vi "Parse and Replace Strings for Downlink.vi"(9 "Input String":string) -> (2 "Output String":string)   [LabVIEW 2010]
doc: "This VI Replaces the string \"ProgramDisabled=YES\" with \"ProgramDisabled=0\" and replaces all instances of \"YES\" with \"1\", all instances of \"NO\" with \"0\". The resulting string is output to the Output String indicator."
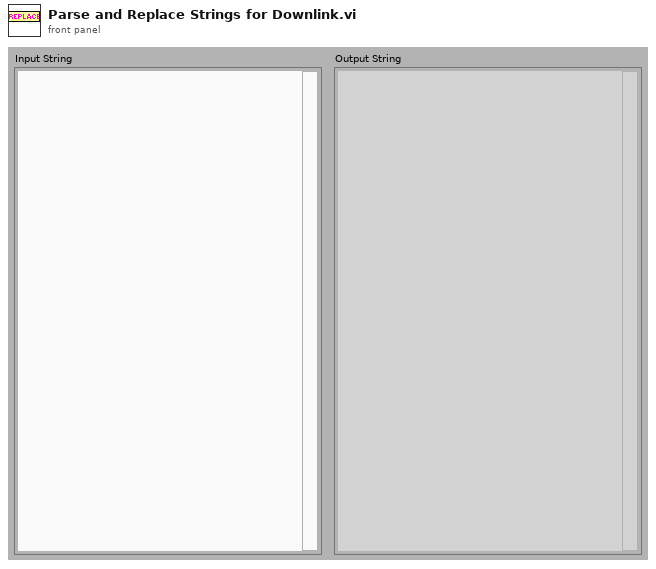
[diagram p1: front panel]
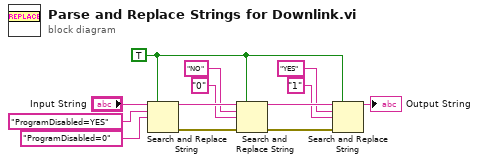
[diagram p0: block diagram]
diagram:
  w7 = TRUE ("replace all? (F)")
  n1 = Search and Replace String(replace all?=w7, input string="Input String", search string="ProgramDisabled=YES" ("regular expression"), replace string="ProgramDisabled=0" ("regular expression")) -> (result string=w13:string, error out=w6:errorcluster)  [unwired: 4 in, 2 out]
  n2 = Search and Replace String(replace all?=w7, input string=w13, search string="NO" ("regular expression"), replace string="0" ("regular expression"), error in=w6) -> (result string=w12:string, error out=w5:errorcluster)  [unwired: 3 in, 2 out]
  n3 = Search and Replace String(replace all?=w7, input string=w12, search string="YES" ("regular expression"), replace string="1" ("regular expression"), error in=w5) -> (result string=→"Output String":string)  [unwired: 3 in, 3 out]
